vi "Pass Fail Check.vi"(6 "Target Rate":dbl, 7 "% tolerance":dbl, 8 "error in (no error)":errorcluster, 11 "WorkspaceManager in":T1) -> (0 "error out":errorcluster, 2 "Possible Failure Modes":bool[](array[boolean]), 3 "WorkspaceManager out":T1)   [LabVIEW 2020]
uses:
  <vilib>/NI VeriStand/Execution/Workspace/WorkspaceAPI.ctl
  NationalInstruments.VeriStand.ClientAPI
  <vilib>/NI VeriStand/Execution/Workspace/NI VeriStand - Get Multiple Channel Values.vi
  <vilib>/regexp/Match Regular Expression.xnode
  <vilib>/NI VeriStand/Execution/Workspace/NI_VS Workspace ExecutionAPI.lvlib
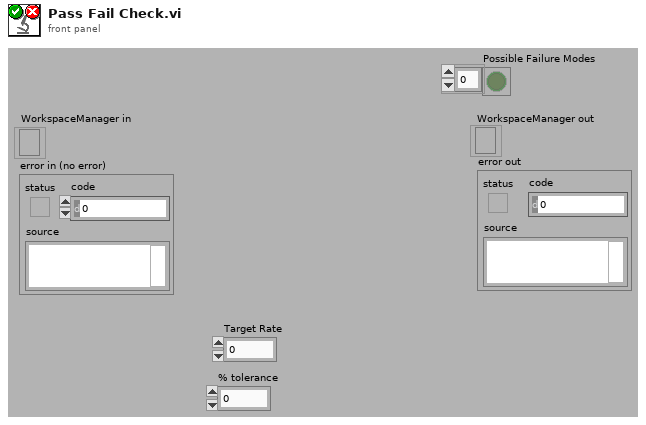
[diagram p1: front panel]
types:
  T1 = typedef "NI_VS Workspace ExecutionAPI.lvlib/WorkspaceAPI.ctl" = refnum<k24>
  T2 = typedef "NI_VS Workspace ExecutionAPI.lvlib/NodeInfo.ctl" = cluster{"Name":string, "FullPath":string, "Type":string, "IsChannel":bool, "Channel":cluster{"Unit":string, "Readable":bool, "Writable":bool, "Faultable":bool, "Scalable":bool, "RowDim":u32, "ColumnDim":u32, "Value Table Names":string[], "Value Table Values":dbl[]}, "IsWaveform":bool, "Waveform":cluster{"DataType":T3}}
  T3 = typedef "NI_VS Workspace ExecutionAPI.lvlib/Waveform Data Type.ctl" = enum16{"Double", "ComplexDouble"}
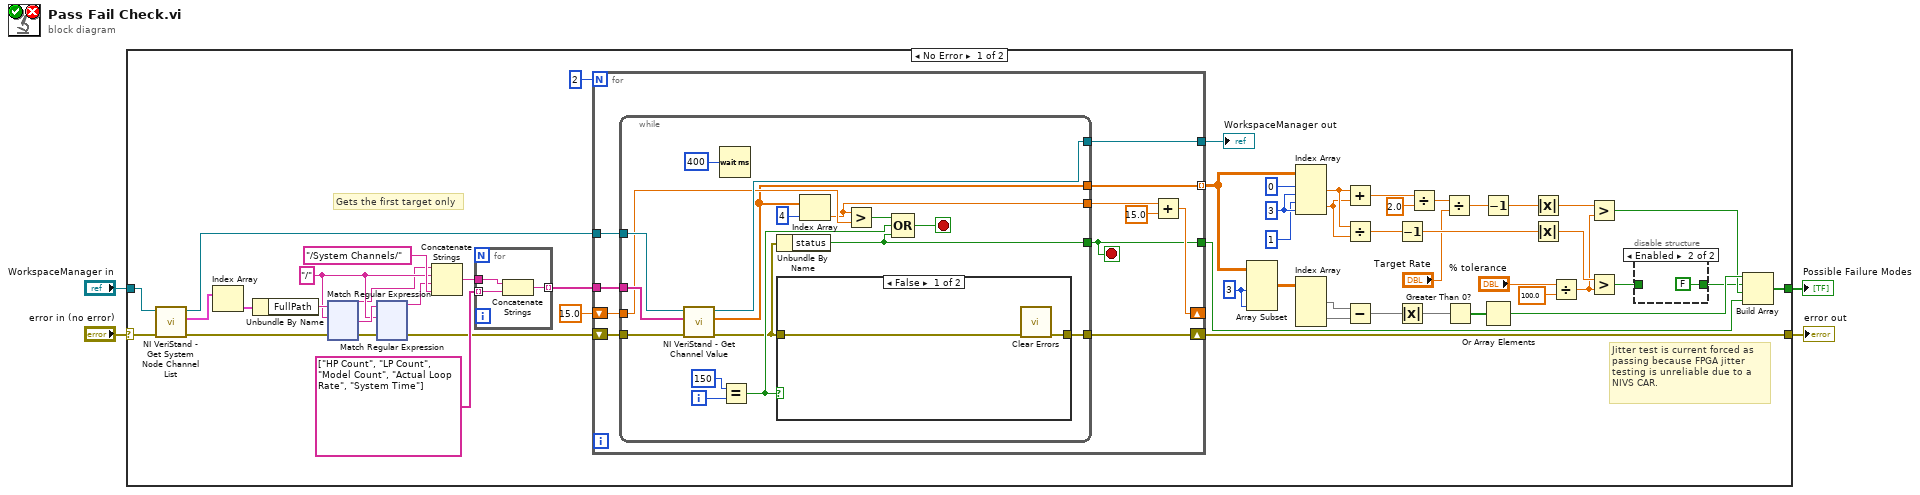
[diagram p0: block diagram]
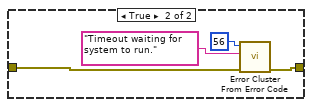
[diagram p3: hidden frame]
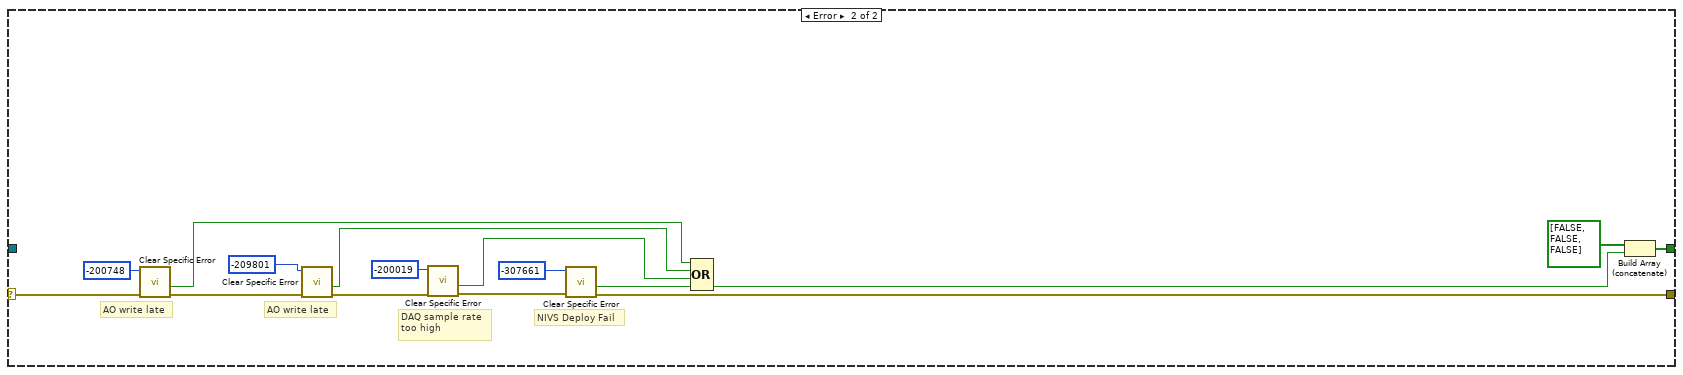
[diagram p4: hidden frame]
diagram:
  n1 = case shown="No Error" "error in (no error)" {
    selector: "error in (no error)" -> [w18 w321]
    tunnel: [w17 w331] -> w2
    tunnel: "WorkspaceManager in" -> [w45 _]
    tunnel: [w14 w330] -> w1
    frame No Error {
      w37 = 3 ("disabled index (col)")
      w41 = 3 ("length")
      w8 = "/" ("format string")
      # "Jitter test is current forced as passing because FPGA jitter testing is unreliable due to a NIVS CAR."
      # "Gets the first target only"
      n2 = call <vilib>:"NI VeriStand - Get System Node Channel List.vi"("error in (no error)"=w18, "WorkspaceManager in"=w45) -> ("error out"=w53:errorcluster, "Channels"=w55:T2[], "WorkspaceManager out"=w48:T1)  [unwired: 7 in]
      n3 = Index Array(array=w55) -> (element=w56:T2)  [unwired: 1 in]
      n4 = Unbundle By Name(w56) -> ("FullPath"=w54:string)
      n5 = xnode "Match Regular Expression"("input string"=w54, "regular expression"=w8, "error in"=w53) -> ("before match"=w7:string, "after match"=w10:string, "error out"=w12:errorcluster)  [unwired: 3 in, 2 out]
      n6 = xnode "Match Regular Expression"("input string"=w10, "regular expression"=w8, "error in"=w12) -> ("before match"=w9:string, "error out"=w11:errorcluster)  [unwired: 3 in, 3 out]
      n7 = Concatenate Strings(w7, w8, w9, "/System Channels/" ("string")) -> (w51:string)
      n8 = for {
        tunnel: w51 -> [w207]
        tunnel: string[] ["HP Count", "LP Count", "Model Count", "Actual Loop Rate", "System Time"] -> [w206] mode=indexing
        tunnel: [w205] -> w49 mode=indexing
        n9 = Concatenate Strings(w207, w206) -> (w205:string)
      }
      n10 = for {
        N: 2 -> [_]
        tunnel: [w180] -> w57
        tunnel: w49 -> [w178]
        tunnel: w48 -> [w177]
        shift-right: [w181] -> w17
        shift-left: w11 -> [w179]
        shift-right: [w173] -> _
        shift-left: 15.0 -> [w176]
        tunnel: [w175] -> w19 mode=indexing
        tunnel: [w171] -> w13
        stop <- w171 stop-if-true
        n11 = while {
          tunnel: [w197] -> w180
          tunnel: [w190] -> w181
          tunnel: w179 -> [w196]
          tunnel: w178 -> [w195]
          tunnel: w177 -> [w194]
          tunnel: w176 -> [w186]
          tunnel: [w185] -> w175
          tunnel: [w184] -> w172
          tunnel: [w182] -> w171
          i -> [w192]
          stop <- w189 stop-if-true
          n12 = call-poly <vilib>:"NI VeriStand - Get Channel Value.vi"("error in (no error)"=w196, "Channels"=w195, "WorkspaceManager in"=w194) -> ("error out"=w183:errorcluster, "Values"=w185:dbl[], "WorkspaceManager out"=w197:T1)  [unwired: 6 in]
          n13 = Wait (ms)(milliseconds to wait=u32 400) -> ()  [unwired: 1 out]
          n14 = Equal?(x=150, y=w192) -> (x = y?=w188:bool)
          n15 = Unbundle By Name(w183) -> ("status"=w182:bool)
          n16 = case shown="False" w188 {
            tunnel: [w199 w203] -> w190
            tunnel: w183 -> [w200 w204]
            frame False {
              n17 = call <vilib>:"Clear Errors.vi"("error in (no error)"=w200) -> ("error out"=w199:errorcluster)  [unwired: 5 in, 1 out]
            }
            frame True {
              n18 = call <vilib>:"Error Cluster From Error Code.vi"("error in (no error)"=w204, "error message (\"\")"="Timeout waiting for system to run." ("error message (\"\")"), "error code (0)"=56) -> ("error out"=w203:errorcluster)  [unwired: 6 in]
            }
          }
          n19 = Index Array(array=w185, index=4) -> (element=w184:dbl)
          n20 = Greater?(x=w184, y=w186) -> (0:w187:bool)
          n21 = Compound Arithmetic op=OR(w187, w188, w182) -> (w189:bool)
        }
        n22 = Add(x=w172, y=15.0) -> (x+y=w173:dbl)
      }
      "WorkspaceManager out" <- w57
      n23 = Array Subset(array=w19, length (row)=w41, length (col)=w41) -> (w42:dbl[][])  [unwired: 2 in]
      n24 = Index Array(array=w19, index (row) #1=0 ("disabled index (row)"), index (col) #1=w37, index (row) #2=1 ("disabled index (row)"), index (col) #2=w37) -> (element #1=w29:dbl, element #2=w28:dbl)
      n25 = Index Array(array=w42) -> (element #1=w40:dbl[], element #2=w39:dbl[])  [unwired: 4 in]
      n26 = Add(x=w29, y=w28) -> (x+y=w27:dbl)
      n27 = Divide(x=w29, y=w28) -> (x/y=w34:dbl)
      n28 = Subtract(x=w40, y=w39) -> (x-y=w43:dbl[])
      n29 = Decrement(x=w34) -> (x-1=w30:dbl)
      n30 = Absolute Value(x=w43) -> (abs(x)=w38:dbl[])
      n31 = Divide(x=w27, y=2.0) -> (x/y=w25:dbl)
      n32 = Divide(x=w25, y="Target Rate") -> (x/y=w23:dbl)
      n33 = Greater Than 0?(x=w38) -> (x > 0?=w44:bool[])
      n34 = Decrement(x=w23) -> (x-1=w22:dbl)
      n35 = Or Array Elements(Boolean array=w44) -> (logical OR=w16:bool)
      n36 = Absolute Value(x=w22) -> (abs(x)=w21:dbl)
      n37 = Absolute Value(x=w30) -> (abs(x)=w33:dbl)
      n38 = Divide(x="% tolerance", y=100.0 ("x")) -> (x/y=w20:dbl)
      n39 = Greater?(x=w21, y=w20) -> (0:w15:bool)
      n40 = Greater?(x=w33, y=w20) -> (0:w5:bool)
      n41 = disable-structure shown="Enabled" {
        disable-tunnel: [w58 FALSE] -> w6
        disable-tunnel: w5 -> [w58 _]
        frame Disabled {
        }
        frame Enabled {
        }
      }
      n42 = Build Array(w16, w6, w15, w13) -> (w14:bool[])
    }
    frame Error {
      # "AO write late"
      # "AO write late"
      # "NIVS Deploy Fail"
      # "DAQ sample rate\ntoo high"
      n43 = call "Clear Specific Error.vi"("error in (no error)"=w321, "code"=-200748) -> ("error out"=w322:errorcluster, "Cleared?"=w319:bool)  [unwired: 8 in]
      n44 = call "Clear Specific Error.vi"("error in (no error)"=w322, "code"=-209801) -> ("error out"=w325:errorcluster, "Cleared?"=w324:bool)  [unwired: 8 in]
      n45 = call "Clear Specific Error.vi"("error in (no error)"=w325, "code"=-200019) -> ("error out"=w329:errorcluster, "Cleared?"=w326:bool)  [unwired: 8 in]
      n46 = call "Clear Specific Error.vi"("error in (no error)"=w329, "code"=-307661 ("x")) -> ("error out"=w331:errorcluster, "Cleared?"=w332:bool)  [unwired: 8 in]
      n47 = Compound Arithmetic op=OR(w319, w324, w326, w332) -> (w328:bool)
      n48 = Build Array (concatenate)(bool[] [FALSE, FALSE, FALSE], w328) -> (w330:bool[])
    }
  }
  "error out" <- w2
  "Possible Failure Modes" <- w1
